vi "Disable.vi"(8 "error in (no error)":errorcluster, 10 "Model in":refnum<class "Model.lvclass">, 11 "Enabled State in":refnum<class "Enabled State.lvclass">) -> (0 "error out":errorcluster, 2 "Model out":refnum<class "Model.lvclass">, 3 "Enabled State out":refnum<class "Enabled State.lvclass">)   [LabVIEW 2015, in "Enabled State.lvclass"]
uses:
  Enabled State.lvclass
  Model/Model/Model.lvclass
  Typedefs/StateTypes.ctl
  Typedefs/FAMT Typedefs.lvlib
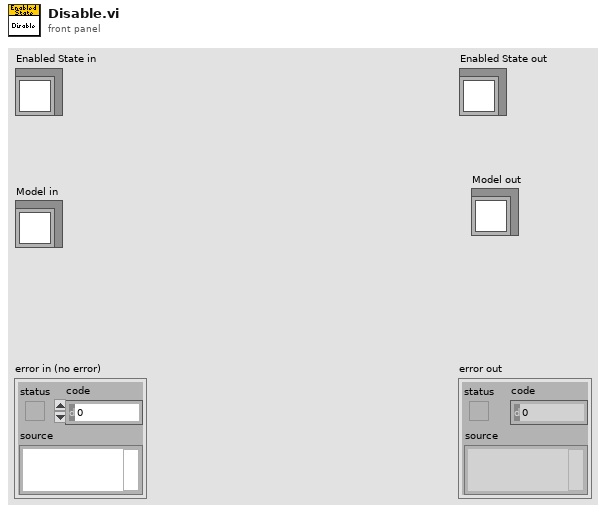
[diagram p1: front panel]
types:
  T1 = typedef "FAMT Typedefs.lvlib/StateTypes.ctl" = enum16{"Offline State", "Fault State", "Standby State", "Disabled State", "Enabled State", "Wait For User Input State", "Test Actuator State"}
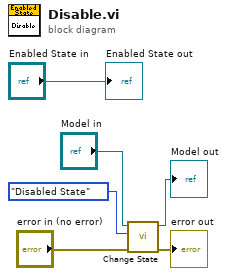
[diagram p0: block diagram]
diagram:
  n1 = call "Change State.vi"("error in (no error)"="error in (no error)", "State Types"=StateTypes."Disabled State" ("State:"), "Model in"="Model in") -> ("error out"=→"error out":errorcluster, "Model out"=→"Model out":refnum<class "Model.lvclass">)  [unwired: 7 in]
  "Enabled State out" <- "Enabled State in"
